vi "WPI_DigitalOutputPulse.vi"(8 "error in (no error)":errorcluster, 10 "length (Sec)":sgl=1.5e-05, 11 "DigitalOutputDevRef":T1={"DIO Channel"=enum."DIO 1", "DevStatus"={"status"=FALSE, "code"=0, "source"=""}}) -> (0 "error out":errorcluster, 3 "DigitalOutputDevRef":T1={"DIO Channel"=enum."DIO 1", "DevStatus"={"status"=FALSE, "code"=0, "source"=""}})   [LabVIEW 2017]
doc: "Emits a hardware-timed pulse for a duration that you specify. For example, you can use this VI to emit a ping from an ultrasonic sensor. This VI sets the value of the digital output to the opposite of the current value. You can use the SetValue VI to specify the starting value of the digital output before you use the Pulse VI.\n\nThis software is licensed. Open the labview\\readme\\WPI Robotics Library Open Source License.txt file for more information."
uses:
  <vilib>/Rock Robotics/WPI/DigitalOutput/WPI_DigitalOutputDevRef.ctl
  <vilib>/Rock Robotics/SystemInterfaces/DIO/FPGA_DIOChannel.ctl
  <vilib>/Rock Robotics/WPI/DigitalModule/WPI_DigitalModuleDIOCacheOp.ctl
  <vilib>/Rock Robotics/SystemInterfaces/System/FPGA_SystemGet.vi
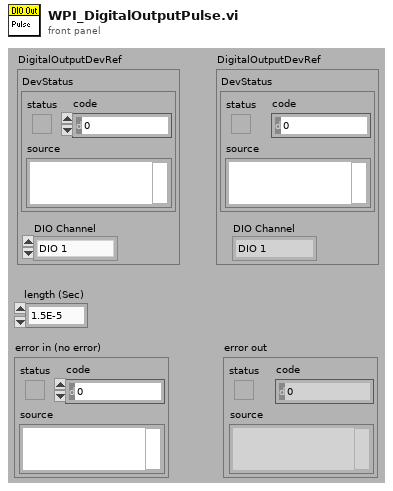
[diagram p1: front panel]
types:
  T1 = typedef "WPI_DigitalOutputDevRef.ctl" = cluster{"DIO Channel":T2, "DevStatus":errorcluster}
  T2 = typedef "FPGA_DIOChannel.ctl" = enum8{"DIO 0", "DIO 1", "DIO 2", "DIO 3", "DIO 4", "DIO 5", "DIO 6", "DIO 7", "DIO 8", "DIO 9", "DIO MXP 0", "DIO MXP 1", "DIO MXP 2", "DIO MXP 3", "DIO MXP 4", "DIO MXP 5", "DIO MXP 6", "DIO MXP 7", "DIO MXP 8", "DIO MXP 9", "DIO MXP 10", "DIO MXP 11", "DIO MXP 12", "DIO MXP 13", "DIO MXP 14", "DIO MXP 15", "SPI Port CS1", "SPI Port CS2", "SPI Port CS3", "SPI Port MISO", "SPI Port MOSI", "Invalid"}
  T3 = typedef "WPI_DigitalModuleDIOCacheOp.ctl" = enum16{"Acquire", "Release", "Status"}
  T4 = typedef "FPGA_DIODevRef.ctl" = cluster{"DevStatus":errorcluster}
  T5 = typedef "WPI_DigitalModuleDeviceRef.ctl" = cluster{"DevStatus":errorcluster}
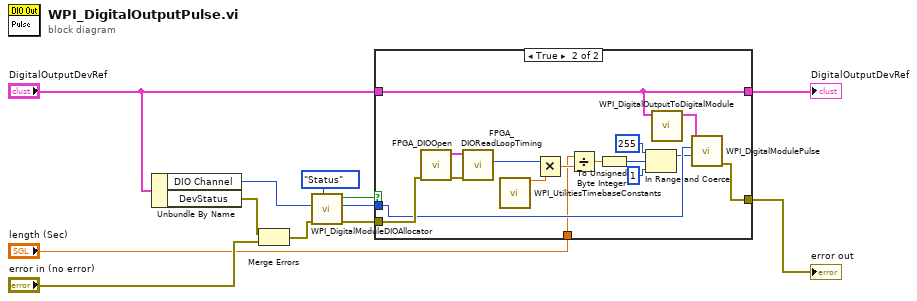
[diagram p0: block diagram]
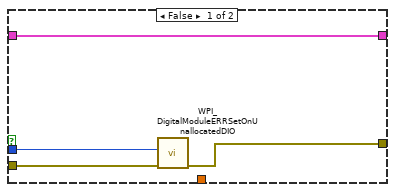
[diagram p2: hidden frame]
diagram:
  n1 = Unbundle By Name("DigitalOutputDevRef") -> ("DIO Channel"=w9:T2, "DevStatus"=w5:errorcluster)
  n2 = Merge Errors(w5, "error in (no error)") -> (w4:errorcluster)
  n3 = call <vilib>:"WPI_DigitalModuleDIOAllocator.vi"("AllocatedDIOMutex"=WPI_DigitalModuleDIOCacheOp."Status", "error in (no error)"=w4, "DIOChannel"=w9) -> ("error out"=w6:errorcluster, "Allocated DIOChannel"=w8:T2, "AllocatedDIO"=w7:bool)  [unwired: 1 in, 5 out]
  n4 = case shown="True" w7 {
    tunnel: "length (Sec)" -> [_ w19]
    tunnel: [w15 w24] -> w3
    tunnel: w8 -> [w14 w25]
    tunnel: w6 -> [w16 w32]
    tunnel: [w13 w17] -> w2
    tunnel: "DigitalOutputDevRef" -> [w13 w17]
    frame False {
      n5 = call <vilib>:"WPI_DigitalModuleERRSetOnUnallocatedDIO.vi"("error in (no error)"=w16, "DIOChannel"=w14) -> ("error out"=w15:errorcluster)  [unwired: 9 in]
    }
    frame True {
      n6 = call <vilib>:"FPGA_DIOOpen.vi"("error in (no error)"=w32) -> ("error out"=w30:errorcluster, "DIODeviceRef"=w31:T4)  [unwired: 1 in, 8 out]
      n7 = call <vilib>:"FPGA_DIOReadLoopTiming.vi"("error in (no error)"=w30, "DIODeviceRef In"=w31) -> ("LoopTiming"=w29:u16)  [unwired: 9 out]
      n8 = call <vilib>:"WPI_UtilitiesTimebaseConstants.vi"() -> ("40 MHz FPGA clock"=w18:dbl)  [unwired: 13 in, 2 out]
      n9 = Multiply(x=w29, y=w18) -> (x*y=w28:dbl)
      n10 = Divide(x=w19, y=w28) -> (x/y=w27:dbl)
      n11 = To Unsigned Byte Integer(number=w27) -> (unsigned 8bit integer=w20:u8)
      n12 = In Range and Coerce(upper limit=u8 255, x=w20, lower limit=u8 1) -> (coerced(x)=w23:u8)  [unwired: 1 out]
      n13 = call <vilib>:"WPI_DigitalOutputToDigitalModule.vi"("DigitalOutputDevRef"=w17) -> ("DigitalModuleDevRef"=w26:T5)  [unwired: 10 out]
      n14 = call <vilib>:"WPI_DigitalModulePulse.vi"("PulseLength"=w23, "DIOChannel"=w25, "DigitalModuleDevRef"=w26) -> ("error out"=w24:errorcluster)  [unwired: 1 in, 7 out]
    }
  }
  "DigitalOutputDevRef" <- w2
  "error out" <- w3
